vi "IMU Loop.vi"(8 "error in (no error)":errorcluster, 11 "FPGA ref in":refnum<k20>) -> (0 "error out":errorcluster)   [LabVIEW 2016]
uses:
  Typedef/INS Data.ctl
  <vilib>/Utility/error.llb/Error Cluster From Error Code.vi
  <vilib>/RVI Host/nirviSupport.llb/nirviErrorClusterFromErrorCode.vi
  <vilib>/rvi/errors/niLvFpgaAdjustHostInterfaceError.vi
  <vilib>/rvi/interface/nirviMethod/nirviMethod.xnode
  <vilib>/ErrorRing/Error Ring.xnode
  <vilib>/rvi/interface/nirviMethod/StockFPGA_InlinedMethodWaitForSingleIRQ.vi
  <vilib>/FPGAPlugInAG/Dynamic/niLvFpga_WaitOnIrq_Dynamic.vi
  <vilib>/FPGAPlugInAG/Dynamic/niLvFpga_AcknowledgeIrq_Dynamic.vi
panel:
  out "roll":sgl
  out "FPGA ref Out":refnum<k20>
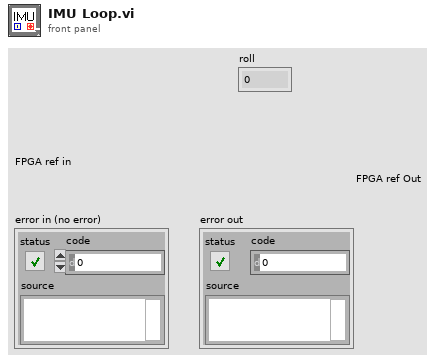
[diagram p1: front panel]
types:
  T1 = typedef "INS Data.ctl" = cluster{"Yaw":sgl, "Pitch":sgl, "Roll":sgl, "Lat":dbl, "Long":dbl, "Alt":dbl, "North":dbl, "East":dbl, "Down":dbl, "PosU":dbl, "VelU":dbl}
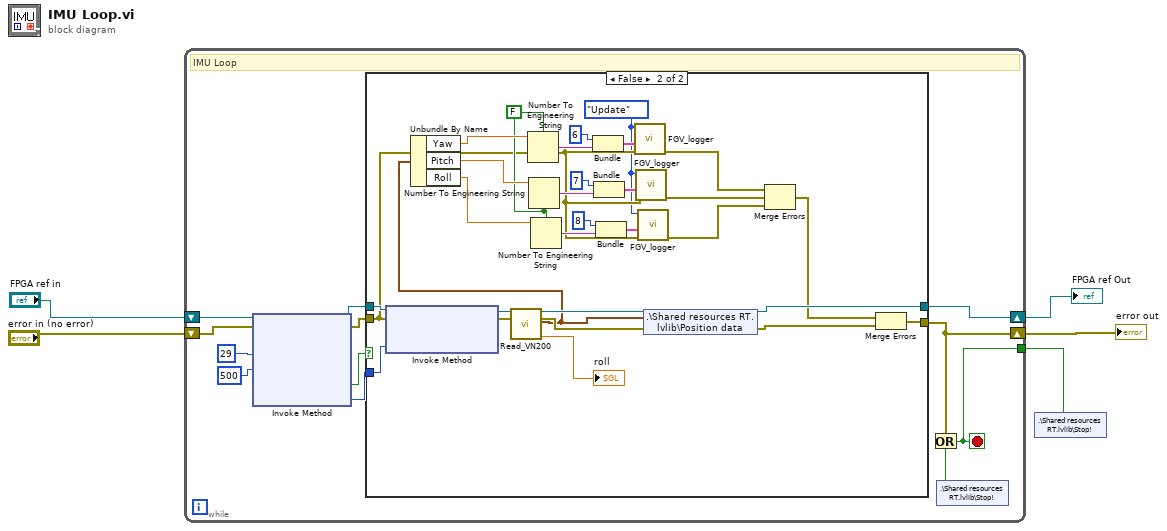
[diagram p0: block diagram]
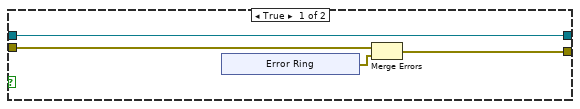
[diagram p2: hidden frame]
diagram:
  n1 = while {
    shift-right: [w15] -> w2
    shift-left: "error in (no error)" -> [w13]
    shift-right: [w17] -> w1
    shift-left: "FPGA ref in" -> [w12]
    tunnel: [w14] -> w3
    stop <- w14 stop-if-true
    # "IMU Loop"
    n2 = xnode "Invoke Method"("FPGA VI Reference In"=w12, "error in"=w13, "IRQ Number(s)"=29, "Timeout (ms)"=500) -> ("FPGA VI Reference Out"=w7:refnum<k20>, "error out"=w8:errorcluster, "Timed Out"=w9:bool, "IRQ(s) Asserted"=w6:i32)
    n3 = case shown="False" w9 {
      tunnel: w8 -> [w20 w35]
      tunnel: w7 -> [w21 w53]
      tunnel: [w21 w55] -> w17
      tunnel: [w19 w49] -> w15
      tunnel: w6 -> [_ w51]
      frame True {
        n4 = xnode "Error Ring"() -> ("error out"=w18:errorcluster)
        n5 = Merge Errors(w20, w18) -> (w19:errorcluster)
      }
      frame False {
        w34 = enum16{"Update", "Log", "Init"}."Update" ("Command")
        w38 = FALSE ("use system decimal point (T)")
        n6 = xnode "Invoke Method"("FPGA VI Reference In"=w53, "error in"=w35, "IRQ Number(s)"=w51) -> ("FPGA VI Reference Out"=w29:refnum<k20>, "error out"=w52:errorcluster)
        n7 = call "Read_VN200.vi"("FPGA Interface"=w29, "error in"=w52) -> ("FPGA Interface Out"=w55:refnum<k20>, "error out"=w54:errorcluster, "Position Data"=w28:T1, "roll"=→"roll":sgl)  [unwired: 10 in]
        n8 = Unbundle By Name(w28) -> ("Yaw"=w45:sgl, "Pitch"=w41:sgl, "Roll"=w37:sgl)
        n9 = Number To Engineering String(1:w38, 4:w45) -> (0:w46:string)  [unwired: 2 in]
        n10 = Number To Engineering String(1:w38, 4:w41) -> (0:w42:string)  [unwired: 2 in]
        n11 = Number To Engineering String(1:w38, 4:w37) -> (0:w39:string)  [unwired: 2 in]
        n12 = Bundle(6, w46) -> (w47:cluster{i32, string})  [unwired: 1 in]
        n13 = Bundle(7, w42) -> (w43:cluster{i32, string})  [unwired: 1 in]
        n14 = Bundle(8, w39) -> (w40:cluster{i32, string})  [unwired: 1 in]
        n15 = call "FGV_logger.vi"("error in"=w35, 9:w47, "Command"=w34) -> ("error out"=w33:errorcluster)  [unwired: 8 in]
        n16 = call "FGV_logger.vi"("error in"=w35, 9:w43, "Command"=w34) -> ("error out"=w32:errorcluster)  [unwired: 8 in]
        n17 = call "FGV_logger.vi"("error in"=w35, 9:w40, "Command"=w34) -> ("error out"=w31:errorcluster)  [unwired: 8 in]
        n18 = shared-variable ".\\Shared resources RT.lvlib\\Position data"(w28, error in=w54) -> (error out=w50:errorcluster)
        n19 = Merge Errors(w33, w32, w31) -> (w30:errorcluster)
        n20 = Merge Errors(w30, w50) -> (w49:errorcluster)
      }
    }
    n21 = shared-variable ".\\Shared resources RT.lvlib\\Stop!"() -> (w16:bool)  [unwired: 1 in, 1 out]
    n22 = Or(x=w15, y=w16) -> (x .or. y?=w14:bool)
  }
  "error out" <- w2
  "FPGA ref Out" <- w1
  n23 = shared-variable ".\\Shared resources RT.lvlib\\Stop!"(w3) -> ()  [unwired: 1 in, 1 out]
